vi "Maps-Set Type.vi"(0 "Google Maps Resource Out in":T1, 7 "Type":string(combo)="hybrid", 11 "error in (no error)":errorcluster) -> (4 "Google Maps Resource Out out":T1, 15 "error out":errorcluster)   [LabVIEW 2020]
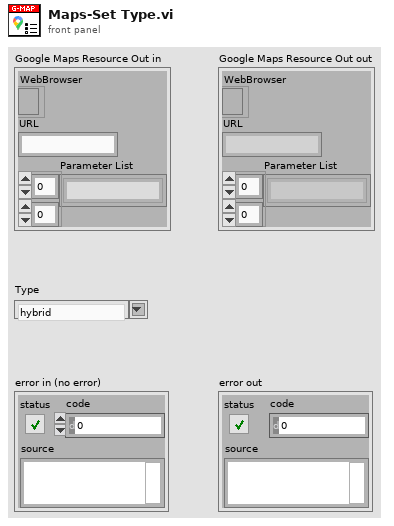
[diagram p1: front panel]
types:
  T1 = cluster{"WebBrowser":refnum<k7>, "URL":string, "Parameter List":string[][]}
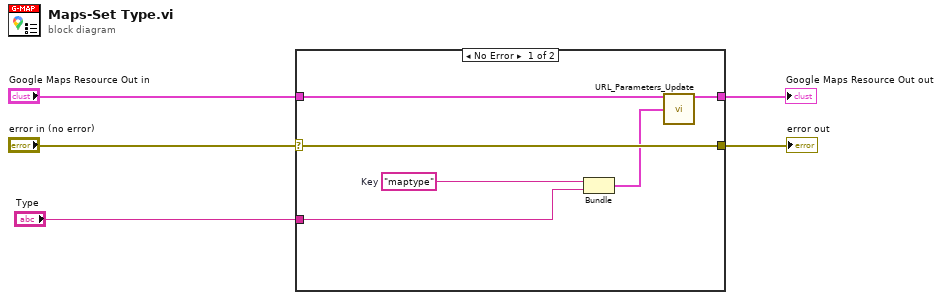
[diagram p0: block diagram]
diagram:
  n1 = case shown="No Error" "error in (no error)" {
    selector: "error in (no error)" -> [w11 w12]
    tunnel: "Google Maps Resource Out in" -> [w9 w13]
    tunnel: [w7 w13] -> w4
    tunnel: [w11 w12] -> w5
    tunnel: "Type" -> [w6 _]
    frame No Error {
      w10 = "maptype"  # Key
      n2 = Bundle("Key"=w10, "Type"=w6) -> (w8:cluster{"Key":string, "Type":string})  [unwired: 1 in]
      n3 = call "URL_Parameters_Update.vi"("Google Maps Resource In"=w9, "URL Parameter"=w8) -> ("Google Maps Resource Out"=w7:T1)  [unwired: 13 in]
    }
    frame Error {
    }
  }
  "error out" <- w5
  "Google Maps Resource Out out" <- w4
